vi "PSK_Image_Transmission.vi"() -> ()   [LabVIEW 2013]
uses:
  <vilib>/picture/picture.llb/Draw True-Color Pixmap.vi
  <vilib>/addons/Modulation/Digital/General/MT Generate PSK System Parameters(M).vi
  <vilib>/addons/Modulation/Digital/General/MT Generate Bits (Galois, PN Order).vi
  <vilib>/addons/Modulation/Digital/General/MT Generate PSK Synchronization Parameters (bit array).vi
  <vilib>/addons/Modulation/Digital/General/MT Format Eye Diagram (complex).vi
  <vilib>/addons/Modulation/niDMT.lvlib
panel:
  out "BER":dbl
  in  "Synchronization Sequence":i32=20
  in  "Zero Pad":i32=16
  out "Sync Found Index":dbl
  out "Error Out":errorcluster
  in  "Stop":bool
  out "Measurements":T1
  in  "Eb/N0 (dB)":dbl(slide)=50.0 scale=-10.0..50.0
  in  "M-PSK":i32=4
  out "Output Bitstream":bool[](array[boolean])
  out "Input Bitstream":bool[](array[boolean])
  out "Baseband Waveform":cluster{"t0":dbl, "dt":dbl, "Y":dbl[]}(graph)
  in  "Tab Control":enum32{"Data", "Constellation", "Eye Diagram"}(tab)
  in  "Scaling Factor":dbl(slide)=5.0 scale=0.0..10.0
  in  "Image File Path":path=path "E:/07/0521/smiley_tiny(recomended).jpg"
  out "Recovered Image":picture
  out "Transmitted Image":picture
  out "Constellation Plot":T2(graph)
  out "Eye Diagram":cluster{"t0":dbl, "dt":dbl, "Y":dbl[]}[](graph)
  # "M-PSK Simulation"
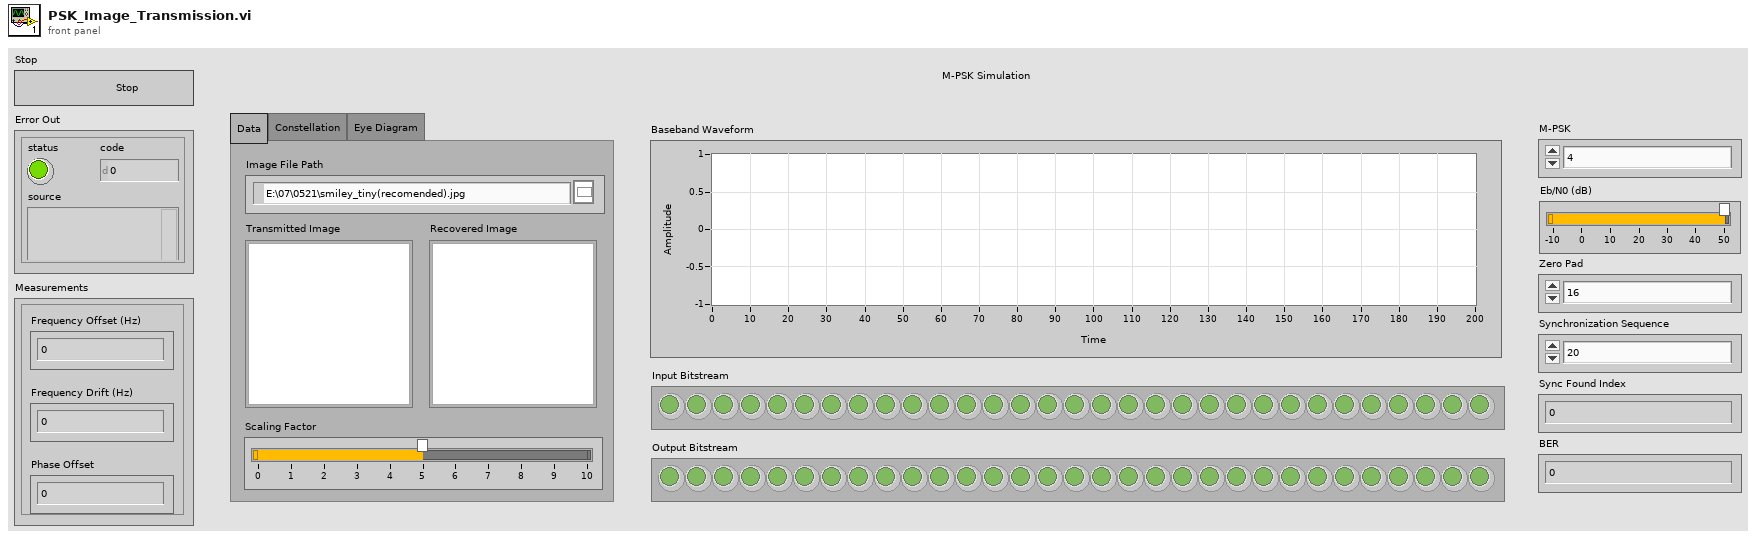
[diagram p1: front panel]
types:
  T1 = cluster{"Frequency Offset (Hz)":dbl, "Frequency Drift (Hz)":dbl, "Phase Offset":dbl}
  T2 = cluster{"constellation":dbl[], "oversampled data":dbl[]}[]
  T3 = typedef "imagedata.ctl" = cluster{"image type":i32, "image depth":i32, "image":u8[], "mask":u8[], "colors":u32[], "Rectangle":cluster{"left":i16, "top":i16, "right":i16, "bottom":i16}}
  T4 = enum16{"FSK", "PSK", "QAM", "MSK", "PAM", "ASK", "CPM"}
  T5 = enum16{"none", "Raised Cosine", "Root Raised Cos", "Gaussian"}
  T6 = cluster{"samples per symbol (16)":i32, "symbol map":cdb[], "differential PSK":enum16{"disable", "enable"}, "PSK type":u16}
  T7 = typedef "niAMT.lvlib/Complex Data Waveform.ctl" = cluster{"t0":dbl, "dt":dbl, "Y":cdb[]}
  T8 = cluster{"expected sync location (symbols)":i32, "sync sequence":cdb[], "sync location uncertainty (symbols)":i32, "sync indent (symbols)":i32}
  T9 = cluster{"frequency offset (Hz)":dbl, "frequency drift (Hz)":dbl, "phase offset (deg)":dbl}
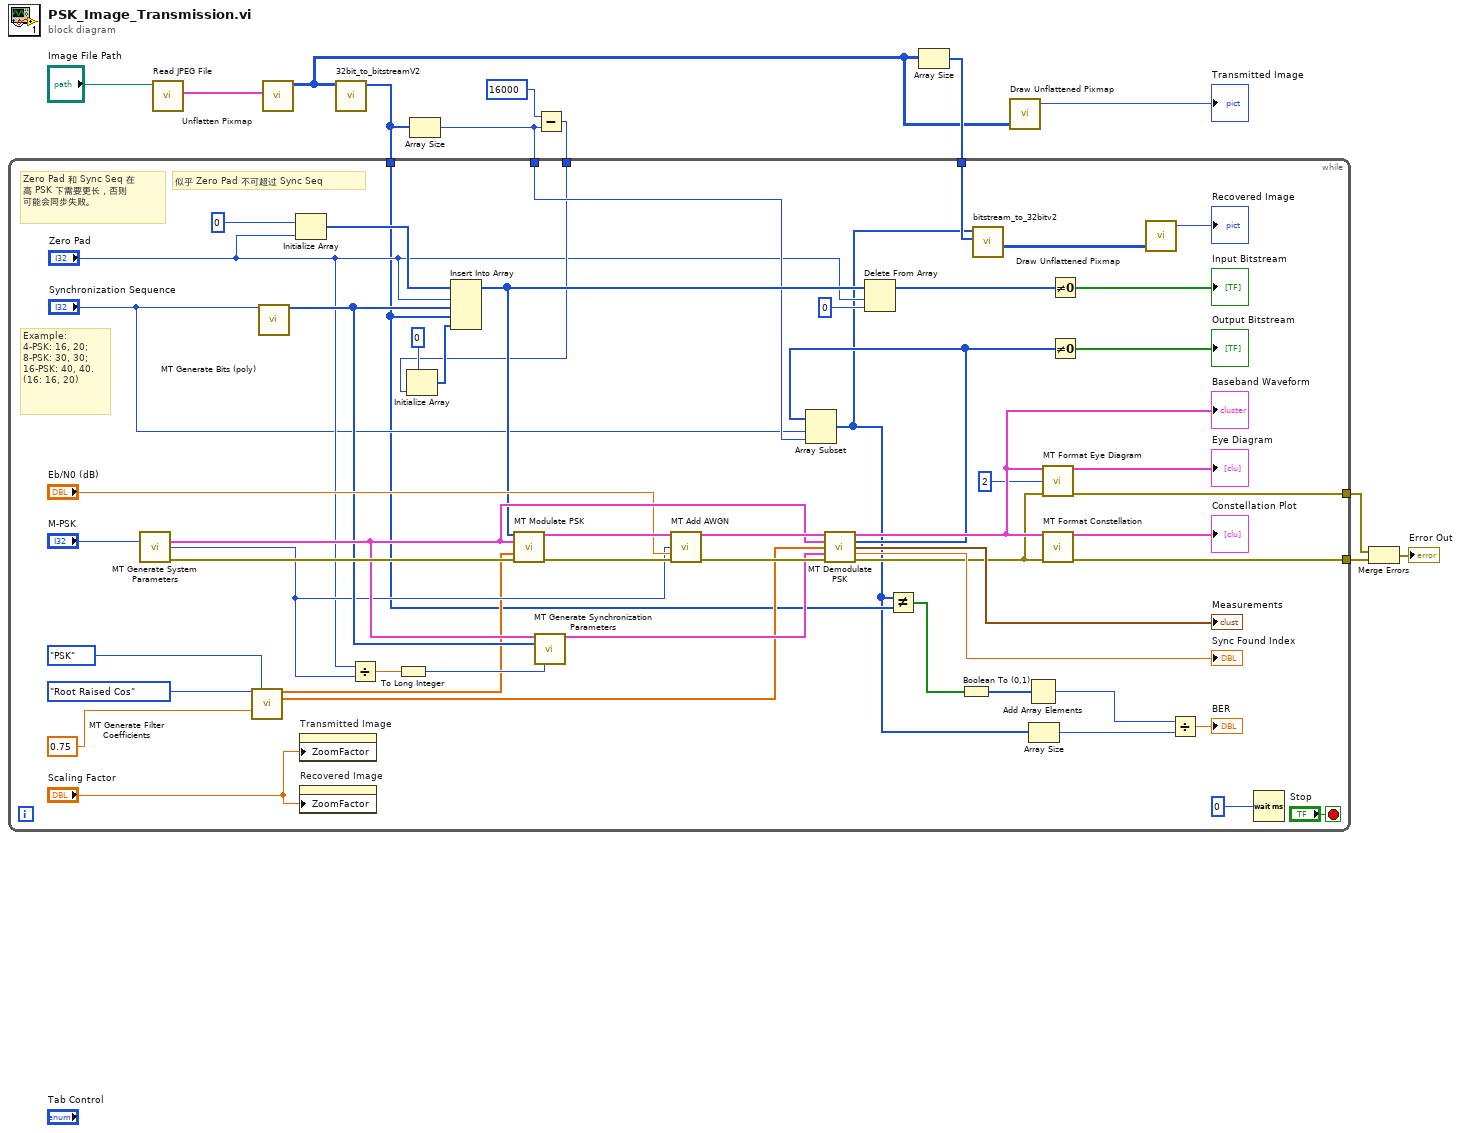
[diagram p0: block diagram]
diagram:
  n1 = call <vilib>:"Read JPEG File.vi"("path to JPEG file"="Image File Path") -> ("image data"=w8:T3)  [unwired: 8 in, 2 out]
  n2 = call <vilib>:"Unflatten Pixmap.vi"("image data"=w8) -> ("24-bit pixmap"=w1:u32[][])  [unwired: 4 in, 6 out]
  n3 = call "32bit_to_bitstreamV2.vi"("24-bit pixmap"=w1) -> ("Bitstream with Guard"=w3:u8[])  [unwired: 7 in, 1 out]
  n4 = Array Size(array=w3) -> (size(s)=w4:i32)
  n5 = Subtract(x=16000, y=w4) -> (x-y=w2:i32)
  n6 = Array Size(array=w1) -> (size(s)=w6:i32[])
  n7 = while {
    tunnel: [w39] -> w10
    tunnel: [w38] -> w11
    tunnel: w6 -> [w27]
    tunnel: w4 -> [w26]
    tunnel: w3 -> [w16]
    tunnel: w2 -> [w23]
    stop <- "Stop" stop-if-true
    # "似乎 Zero Pad 不可超过 Sync Seq"
    # "Example:\n4-PSK: 16, 20;\n8-PSK: 30, 30;\n16-PSK: 40, 40.\n(16: 16, 20)"
    # "Zero Pad 和 Sync Seq 在\n高 PSK 下需要更长，否则\n可能会同步失败。"
    n8 = call-poly <vilib>:"MT Generate System Parameters.vi"("M-PSK (4)"="M-PSK") -> ("PSK system parameters"=w48:T6, "bits per symbol"=w42:i32, "error out"=w57:errorcluster)  [unwired: 12 in]
    n9 = call <vilib>:"MT Generate Filter Coefficients.vi"("pulse shaping filter (none)"=T5."Root Raised Cos", "modulation type"=T4."PSK", "filter parameter"=0.75) -> ("pulse shaping filter coefficients"=w36:dbl[], "matched filter coefficients"=w35:dbl[])  [unwired: 10 in, 1 out]
    n10 = call-poly <vilib>:"MT Generate Bits (poly).vi"("total bits (128)"="Synchronization Sequence") -> ("output bit stream"=w43:i8[])  [unwired: 12 in, 2 out]
    n11 = Initialize Array "Initialize Array"(0, "Zero Pad") -> (w64:i32[])
    n12 = property on="Transmitted Image" class="Pict"("ZoomFactor"="Scaling Factor") -> ()  [unwired: 2 in, 2 out]
    n13 = property on="Recovered Image" class="Pict"("ZoomFactor"="Scaling Factor") -> ()  [unwired: 2 in, 2 out]
    n14 = Divide(x="Zero Pad", y=w42) -> (x/y=w45:dbl)
    n15 = To Long Integer(number=w45) -> (32bit integer=w44:i32)
    n16 = Initialize Array "Initialize Array"(0, w23) -> (w24:i32[])
    n17 = Insert Into Array "Insert Into Array"(array=w64, index="Zero Pad", new element #1=w43, new element #2=w16, new element #3=w24) -> (w31:i32[])
    n18 = call <vilib>:"MT Modulate PSK.vi"("input bit stream"=w31, "PSK system parameters"=w48, "pulse shaping filter coefficients"=w36, "error in (no error)"=w57) -> ("output complex waveform"=w56:T7, "error out"=w55:errorcluster)  [unwired: 9 in, 1 out]
    n19 = call-poly <vilib>:"MT Generate Synchronization Parameters.vi"("PSK system parameters"=w48, "sync bits"=w43, "expected sync location (symbols)"=w44) -> ("PSK synchronization parameters"=w47:T8)  [unwired: 11 in, 1 out]
    n20 = call <vilib>:"MT Add AWGN.vi"("input complex waveform"=w56, "bits per symbol (1)"=w42, "Eb/N0 (10 dB)"="Eb/N0 (dB)", "error in (no error)"=w55) -> ("output complex waveform"=w53:T7, "error out"=w54:errorcluster)  [unwired: 9 in, 1 out]
    n21 = call <vilib>:"MT Demodulate PSK.vi"("input complex waveform"=w53, "PSK system parameters"=w48, "matched filter coefficients"=w35, "synchronization parameters"=w47, "error in (no error)"=w54) -> ("recovered complex waveform"=w51:T7, "output bit stream"=w28:i8[], "measurements"=→"Measurements":T9, "sync found index (symbols)"=→"Sync Found Index":dbl, "error out"=w37:errorcluster)  [unwired: 6 in]
    "Baseband Waveform" <- w51
    n22 = Array Subset "Array Subset"(array=w28, index="Synchronization Sequence", length=w26) -> (w13:i8[])
    n23 = Delete From Array "Delete From Array"(array=w31, length="Zero Pad", index=0) -> (array with subset deleted=w63:i32[])  [unwired: 1 out]
    n24 = Not Equal?(x=w13, y=w16) -> (x != y?=w15:bool[])
    n25 = Boolean To (0,1)(Boolean=w15) -> (0, 1=w14:i16[])
    n26 = call "bitstream_to_32bitv2.vi"("JPG Size"=w27, "Bitstream Input"=w13) -> ("2D JPG Array"=w29:u32[][])  [unwired: 8 in, 1 out]
    n27 = Add Array Elements(numeric array=w14) -> (sum=w18:i16)
    n28 = Array Size(array=w13) -> (size(s)=w17:i32)
    n29 = call-poly <vilib>:"MT Format Eye Diagram.vi"("waveform"=w51, "eye length"=2, "error in (no error)"=w37) -> ("eye diagram"=→"Eye Diagram":cluster{"t0":dbl, "dt":dbl, "Y":dbl[]}[], "error out"=w39:errorcluster)  [unwired: 11 in]
    n30 = call <vilib>:"MT Format Constellation.vi"("waveform"=w51, "error in (no error)"=w37) -> ("constellation graph"=→"Constellation Plot":T2, "error out"=w38:errorcluster)  [unwired: 12 in]
    n31 = Not Equal To 0?(x=w63) -> (x != 0?=→"Input Bitstream":bool[])
    n32 = Not Equal To 0?(x=w28) -> (x != 0?=→"Output Bitstream":bool[])
    n33 = call-poly <vilib>:"Draw Unflattened Pixmap.vi"("data (RGB format)"=w29) -> ("new picture"=→"Recovered Image":picture)  [unwired: 8 in]
    n34 = Divide(x=w18, y=w17) -> (x/y=→"BER":dbl)
    n35 = Wait (ms)(milliseconds to wait=0) -> ()  [unwired: 1 out]
  }
  n36 = call-poly <vilib>:"Draw Unflattened Pixmap.vi"("data (RGB format)"=w1) -> ("new picture"=→"Transmitted Image":picture)  [unwired: 8 in]
  n37 = Merge Errors(w10, w11) -> (→"Error Out":errorcluster)
